vi "Total Days in Month.vi"(9 "Year":string(combo), 10 "Month":string(combo)) -> (1 "All Days":string[](array[string]), 2 "Total Days in Month":string)   [LabVIEW 2017]
uses:
  <vilib>/Utility/miscctls.llb/LVDateTimeRec.ctl
panel:
  out "time stamp":timestamp
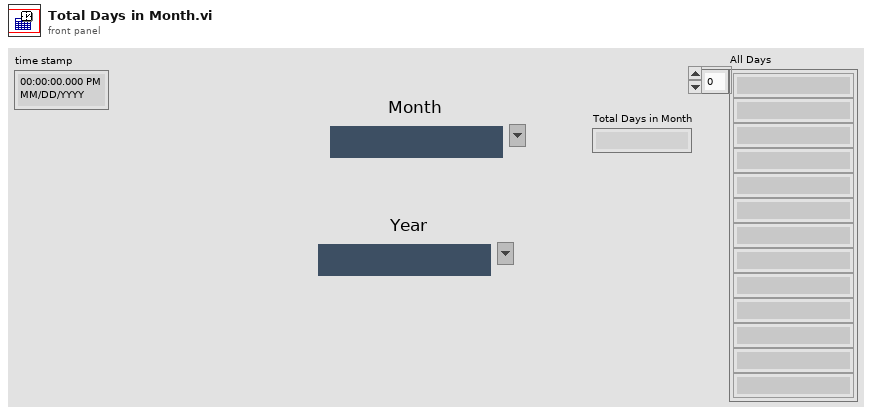
[diagram p1: front panel]
types:
  T1 = typedef "LVDateTimeRec.ctl" = cluster{"fractional second":dbl, "second":i32, "minute":i32, "hour":i32, "day of month":i32, "month":i32, "year":i32, "day of week":i32, "day of year":i32, "DST":i32}
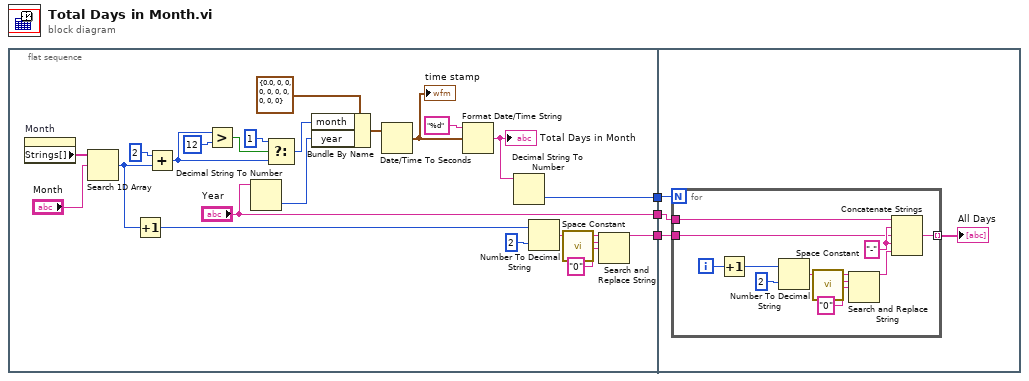
[diagram p0: block diagram]
diagram:
  n1 = flat-sequence {
    tunnel: [w13] -> w3
    tunnel: ["Year"] -> w2
    tunnel: [w5] -> w1
    tunnel: w3 -> [w30]
    tunnel: w2 -> [w29]
    tunnel: w1 -> [w28]
    frame #0 {
      n2 = property on="Month" class="CmbBox"() -> ("Strings[]"=w12:string[])  [unwired: 2 in, 2 out]
      n3 = Search 1D Array(1D array=w12, element="Month") -> (index of element=w11:i32)  [unwired: 1 in]
      n4 = Increment(x=w11) -> (x+1=w10:i32)
      n5 = Add(x=2, y=w11) -> (x+y=w18:i32)
      n6 = Greater?(x=w18, y=12) -> (0:w19:bool)
      n7 = Decimal String To Number(string="Year") -> (number=w15:i32)  [unwired: 2 in, 1 out]
      n8 = Select(t=1, s=w19, f=w18) -> (s? t:f=w16:i32)
      n9 = Bundle By Name(cluster=T1 {"fractional second"=0.0, "second"=0, "minute"=0, "hour"=0, "day of month"=0, "month"=0, "year"=0, "day of week"=0, "day of year"=0, "DST"=0} ("date time rec"), "month"=w16, "year"=w15) -> (w26:T1)
      n10 = Date/Time To Seconds(2:w26) -> (0:w24:timestamp)  [unwired: 1 in]
      "time stamp" <- w24
      n11 = Format Date/Time String(time format string (%c)="%d", seconds (now)=w24) -> (date/time string=w14:string)  [unwired: 1 in]
      "Total Days in Month" <- w14
      n12 = Decimal String To Number(string=w14) -> (number=w13:i32)  [unwired: 2 in, 1 out]
      n13 = Number To Decimal String(number=w10, width (-)=i16 2) -> (decimal integer string=w8:string)
      n14 = call <vilib>:"Space Constant.vi"() -> ("String"=w7:string)
      n15 = Search and Replace String(input string=w8, search string=w7, replace string="0" ("replace string (\"\")")) -> (result string=w5:string)  [unwired: 5 in, 3 out]
    }
    frame #1 {
      n16 = for {
        N: w30 -> [_]
        tunnel: w29 -> [w39]
        tunnel: w28 -> [w37]
        tunnel: [w36] -> w27 mode=indexing
        i -> [w41]
        w38 = "-"
        n17 = Increment(x=w41) -> (x+1=w40:i32)
        n18 = Number To Decimal String(number=w40, width (-)=i16 2) -> (decimal integer string=w32:string)
        n19 = call <vilib>:"Space Constant.vi"() -> ("String"=w33:string)
        n20 = Search and Replace String(input string=w32, search string=w33, replace string="0" ("replace string (\"\")")) -> (result string=w31:string)  [unwired: 5 in, 3 out]
        n21 = Concatenate Strings(w39, w38, w37, w38, w31) -> (w36:string)
      }
      "All Days" <- w27
    }
  }
